vi "ProtoBuff - Separate Message Size and Message.vi"(9 "Input String":string) -> (1 "Protobuf String Output":string, 2 "Protobuf Message Size":u32)   [LabVIEW 2020]
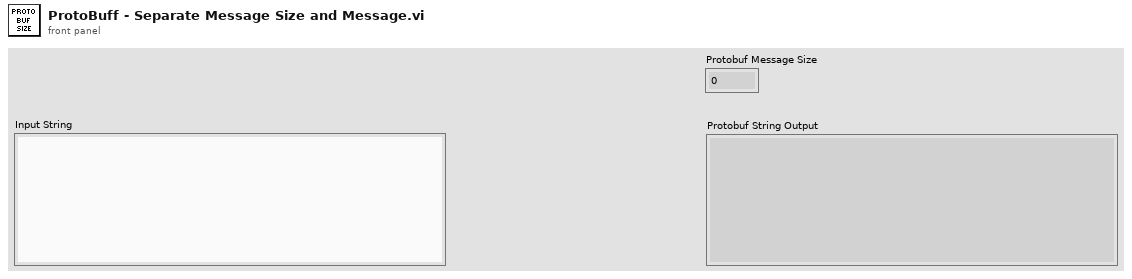
[diagram p1: front panel]
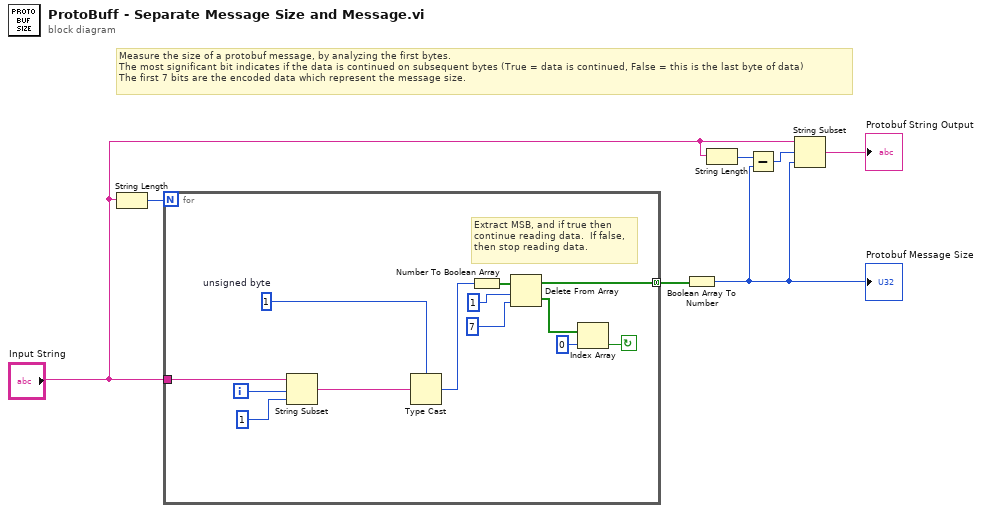
[diagram p0: block diagram]
diagram:
  # "Measure the size of a protobuf message, by analyzing the first bytes.\nThe most significant bit indicates if the data is continued on subsequent bytes (True = data is continued, False = this is the last byte of data)\nThe first 7 bits are the encoded data which represent the message size."
  n1 = String Length(string="Input String") -> (length=w7:i32)
  n2 = for {
    N: w7 -> [_]
    tunnel: [w13] -> w6 mode=concatenating
    tunnel: "Input String" -> [w12]
    i -> [w11]
    stop <- w8 continue-if-true
    w20 = u8 1  # unsigned byte
    # "Extract MSB, and if true then\ncontinue reading data.  If false,\nthen stop reading data."
    n3 = String Subset(string=w12, offset (0)=w11, length (rest)=1 ("length (rest)")) -> (substring=w9:string)
    n4 = Type Cast(type=w20, x=w9) -> (*(type *) &x=w19:u8)
    n5 = Number To Boolean Array(number=w19) -> (Boolean array=w18:bool[])
    n6 = Delete From Array(array=w18, length=1, index=7) -> (deleted portion=w15:bool[], array with subset deleted=w13:bool[])
    n7 = Index Array(array=w15, index=0) -> (element=w8:bool)
  }
  n8 = Boolean Array To Number(Boolean array=w6) -> (number=w2:u32)
  "Protobuf Message Size" <- w2
  n9 = String Length(string="Input String") -> (length=w4:i32)
  n10 = Subtract(x=w4, y=w2) -> (x-y=w1:u32)
  n11 = String Subset(string="Input String", offset (0)=w1, length (rest)=w2) -> (substring=→"Protobuf String Output":string)
